vi "check x mirror speed.vi"() -> (3 "mirror speed valid":bool)   [LabVIEW 2012]
uses:
  GFG/GFGnumericGet.vi
  GFG/GFGbooleanGet.vi
  GFG/GFGfpRefGet.vi
  GFG/GFG library.lvlib
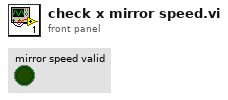
[diagram p1: front panel]
types:
  T1 = cluster{"Boolean":bool, "Numeric":dbl, "Numeric":dbl}
  T2 = cluster{"Boolean":bool, "Numeric":bool, "Numeric":bool}
  T3 = enum8{"Enabled", "Disabled", "Disabled and Grayed Out"}
  T4 = cluster{"WaveformChartRef":refnum<vi>, "DigitalRef":refnum<vi>, "ArrayRef":refnum<vi>, "TabControlRef":refnum<vi>, "EnumRef":refnum<vi>, "RingRef":refnum<vi>, "BooleanRef":refnum<vi>, "KnobRef":refnum<vi>, "SlideRef":refnum<vi>, "PathRef":refnum<vi>, "StringRef":refnum<vi>, "ComboBox":refnum<vi>, "WaveformGraphRef":refnum<vi>}
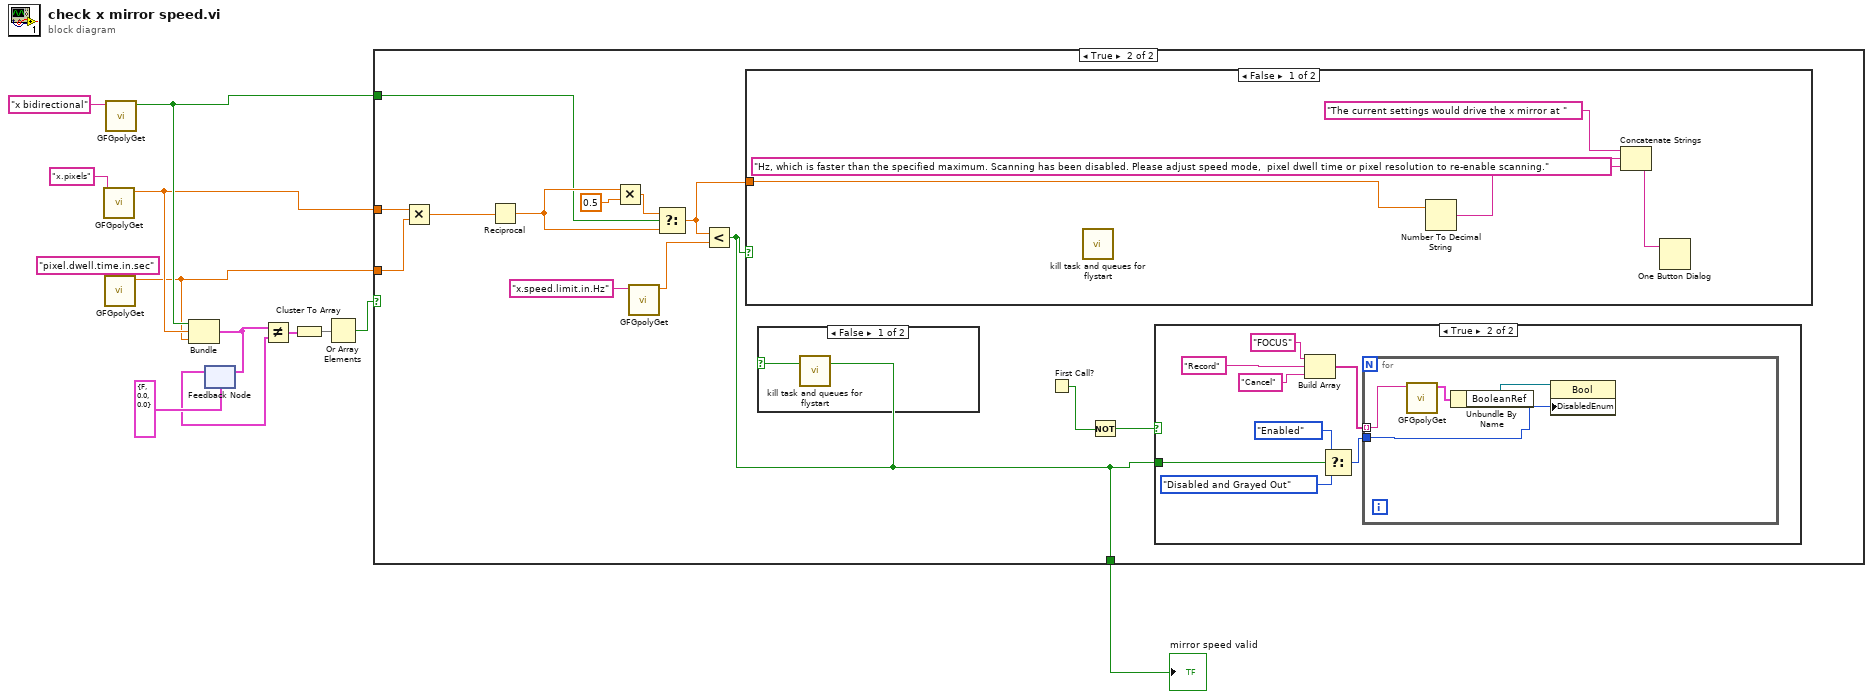
[diagram p0: block diagram]
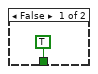
[diagram p2: hidden frame]
diagram:
  n1 = call-poly "GFGpolyGet.vi"("Variable Name in"="x.pixels") -> ("Numeric"=w9:dbl)  [unwired: 9 in, 1 out]
  n2 = call-poly "GFGpolyGet.vi"("Variable Name in"="pixel.dwell.time.in.sec") -> ("Numeric"=w8:dbl)  [unwired: 9 in, 1 out]
  n3 = call-poly "GFGpolyGet.vi"("Variable Name in"="x bidirectional") -> ("Boolean"=w10:bool)  [unwired: 10 in]
  n4 = Bundle("Boolean"=w10, "Numeric"=w9, "Numeric"=w8) -> (w6:T1)  [unwired: 1 in]
  n5 = feedback #1(T1 {"Boolean"=FALSE, "Numeric"=0.0, "Numeric"=0.0}) -> (w5:T1)
  n6 = feedback-in #1(w6) -> ()
  n7 = Not Equal?(x=w6, y=w5) -> (x != y?=w4:T2)
  n8 = Cluster To Array(cluster=w4) -> (array=w2:bool[])
  n9 = Or Array Elements(Boolean array=w2) -> (logical OR=w3:bool)
  n10 = case shown="True" w3 {
    tunnel: w10 -> [_ w22]
    tunnel: w9 -> [_ w20]
    tunnel: w8 -> [_ w19]
    tunnel: [TRUE w17] -> w1
    frame False {
    }
    frame True {
      n11 = Multiply(x=w20, y=w19) -> (x*y=w21:dbl)
      n12 = Reciprocal(x=w21) -> (1/x=w23:dbl)
      n13 = Multiply(x=w23, y=0.5) -> (x*y=w24:dbl)
      n14 = call-poly "GFGpolyGet.vi"("Variable Name in"="x.speed.limit.in.Hz") -> ("Numeric"=w27:dbl)  [unwired: 9 in, 1 out]
      n15 = Select(t=w24, s=w22, f=w23) -> (s? t:f=w18:dbl)
      n16 = Less?(x=w18, y=w27) -> (x < y?=w17:bool)
      n17 = case shown="False" w17 {
        tunnel: w18 -> [w44 _]
        frame False {
          n18 = call "kill task and queues for flystart.vi"() -> ()  [unwired: 12 in]
          n19 = Number To Decimal String(number=w44) -> (decimal integer string=w42:string)  [unwired: 1 in]
          n20 = Concatenate Strings("The current settings would drive the x mirror at " ("message"), w42, "Hz, which is faster than the specified maximum. Scanning has been disabled. Please adjust speed mode,  pixel dwell time or pixel resolution to re-enable scanning." ("string")) -> (w40:string)
          n21 = One Button Dialog(message=w40) -> ()  [unwired: 1 in, 1 out]
        }
        frame True {
        }
      }
      n22 = case shown="False" w17 {
        frame False {
          n23 = call "kill task and queues for flystart.vi"() -> ()  [unwired: 12 in]
        }
        frame True {
        }
      }
      n24 = First Call?() -> (First Call?: T/F=w16:bool)
      n25 = Not(x=w16) -> (.not. x?=w15:bool)
      n26 = case shown="True" w15 {
        tunnel: w17 -> [_ w28]
        frame False {
        }
        frame True {
          n27 = Build Array("FOCUS" ("Variable Name in"), "Record" ("element"), "Cancel" ("element")) -> (w35:string[])
          n28 = Select(t=T3."Enabled" ("Disabled"), s=w28, f=T3."Disabled and Grayed Out" ("Disabled")) -> (s? t:f=w30:T3)
          n29 = for {
            tunnel: w35 -> [w37] mode=indexing
            tunnel: w30 -> [w36]
            n30 = call-poly "GFGpolyGet.vi"("Variable Name in"=w37) -> ("output cluster"=w39:T4)  [unwired: 9 in, 1 out]
            n31 = Unbundle By Name(w39) -> ("BooleanRef"=w38:refnum<vi>)
            n32 = property class="Bool"(reference=w38, "DisabledEnum"=w36) -> ()  [unwired: 1 in, 2 out]
          }
        }
      }
    }
  }
  "mirror speed valid" <- w1
